vi "Digital Inputs Write.vi"(4 "error in (no error)":errorcluster, 5 "Value":string[](array[string]), 6 "Container State":T2, 7 "Display State In":T1) -> (0 "error out":errorcluster, 3 "Display State Out":T1)   [LabVIEW 2015, in "Input Event XCtrl.xctl"]
uses:
  Input Event XCtrl.xctl
  <vilib>/_xctls/Container State.ctl
  State.vi
  <vilib>/_xctls/XControlSupport.lvlib
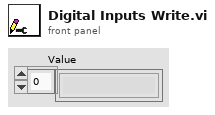
[diagram p1: front panel]
types:
  T1 = typedef "Input Event XCtrl.xctl/State.vi" = cluster{"Digital Inputs":string[], "Flags":string[], "action":string}
  T2 = typedef "XControlSupport.lvlib/Container State.ctl" = cluster{"Indicator?":bool, "Run Mode?":bool, " Refnum":refnum<vi>}
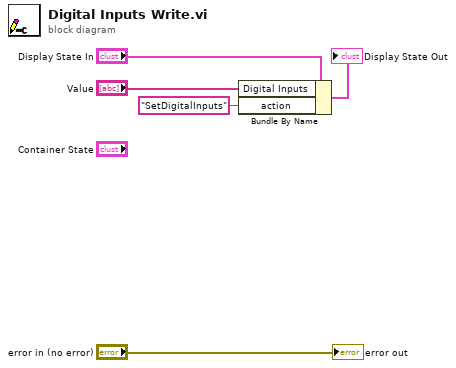
[diagram p0: block diagram]
diagram:
  n1 = Bundle By Name(cluster="Display State In", "Digital Inputs"="Value", "action"="SetDigitalInputs") -> (→"Display State Out":T1)
  "error out" <- "error in (no error)"
